vi "Parse VI Documentation String.vi"(5 "LANG ID":string="CＮ", 7 "NOTE-Map":variant, 11 "Documentation":string) -> (0 "Ctrl-Doc Map":variant, 1 "Control Docs":cluster{"filtered array":string[]}[](array[cluster]), 2 "Core Doc":string, 3 "Documentation (Dup)":string, 4 "OUTPUT":string, 6 "INPUT":string)   [LabVIEW 2017, in "csmdoc.lvlib"]
doc: "### Parse VI Documentation String.vi\n\n-- <b>Controls</b> --\n- <b>NOTE-Map</b>:\n- <b>Documentation</b>:\n\n-- <b>Indicators</b> --\n- <b>Ctrl-Doc Map</b>:\n- <b>Control Docs</b>:\n- <b>Core Doc</b>:\n- <b>Documentation (dup)</b>:"
uses:
  csmdoc.lvlib
  _tool/_file/csm-file-support.lvlib
  Communicable State Machine.lvlib
  _Shared/CSM Shared.lvlib
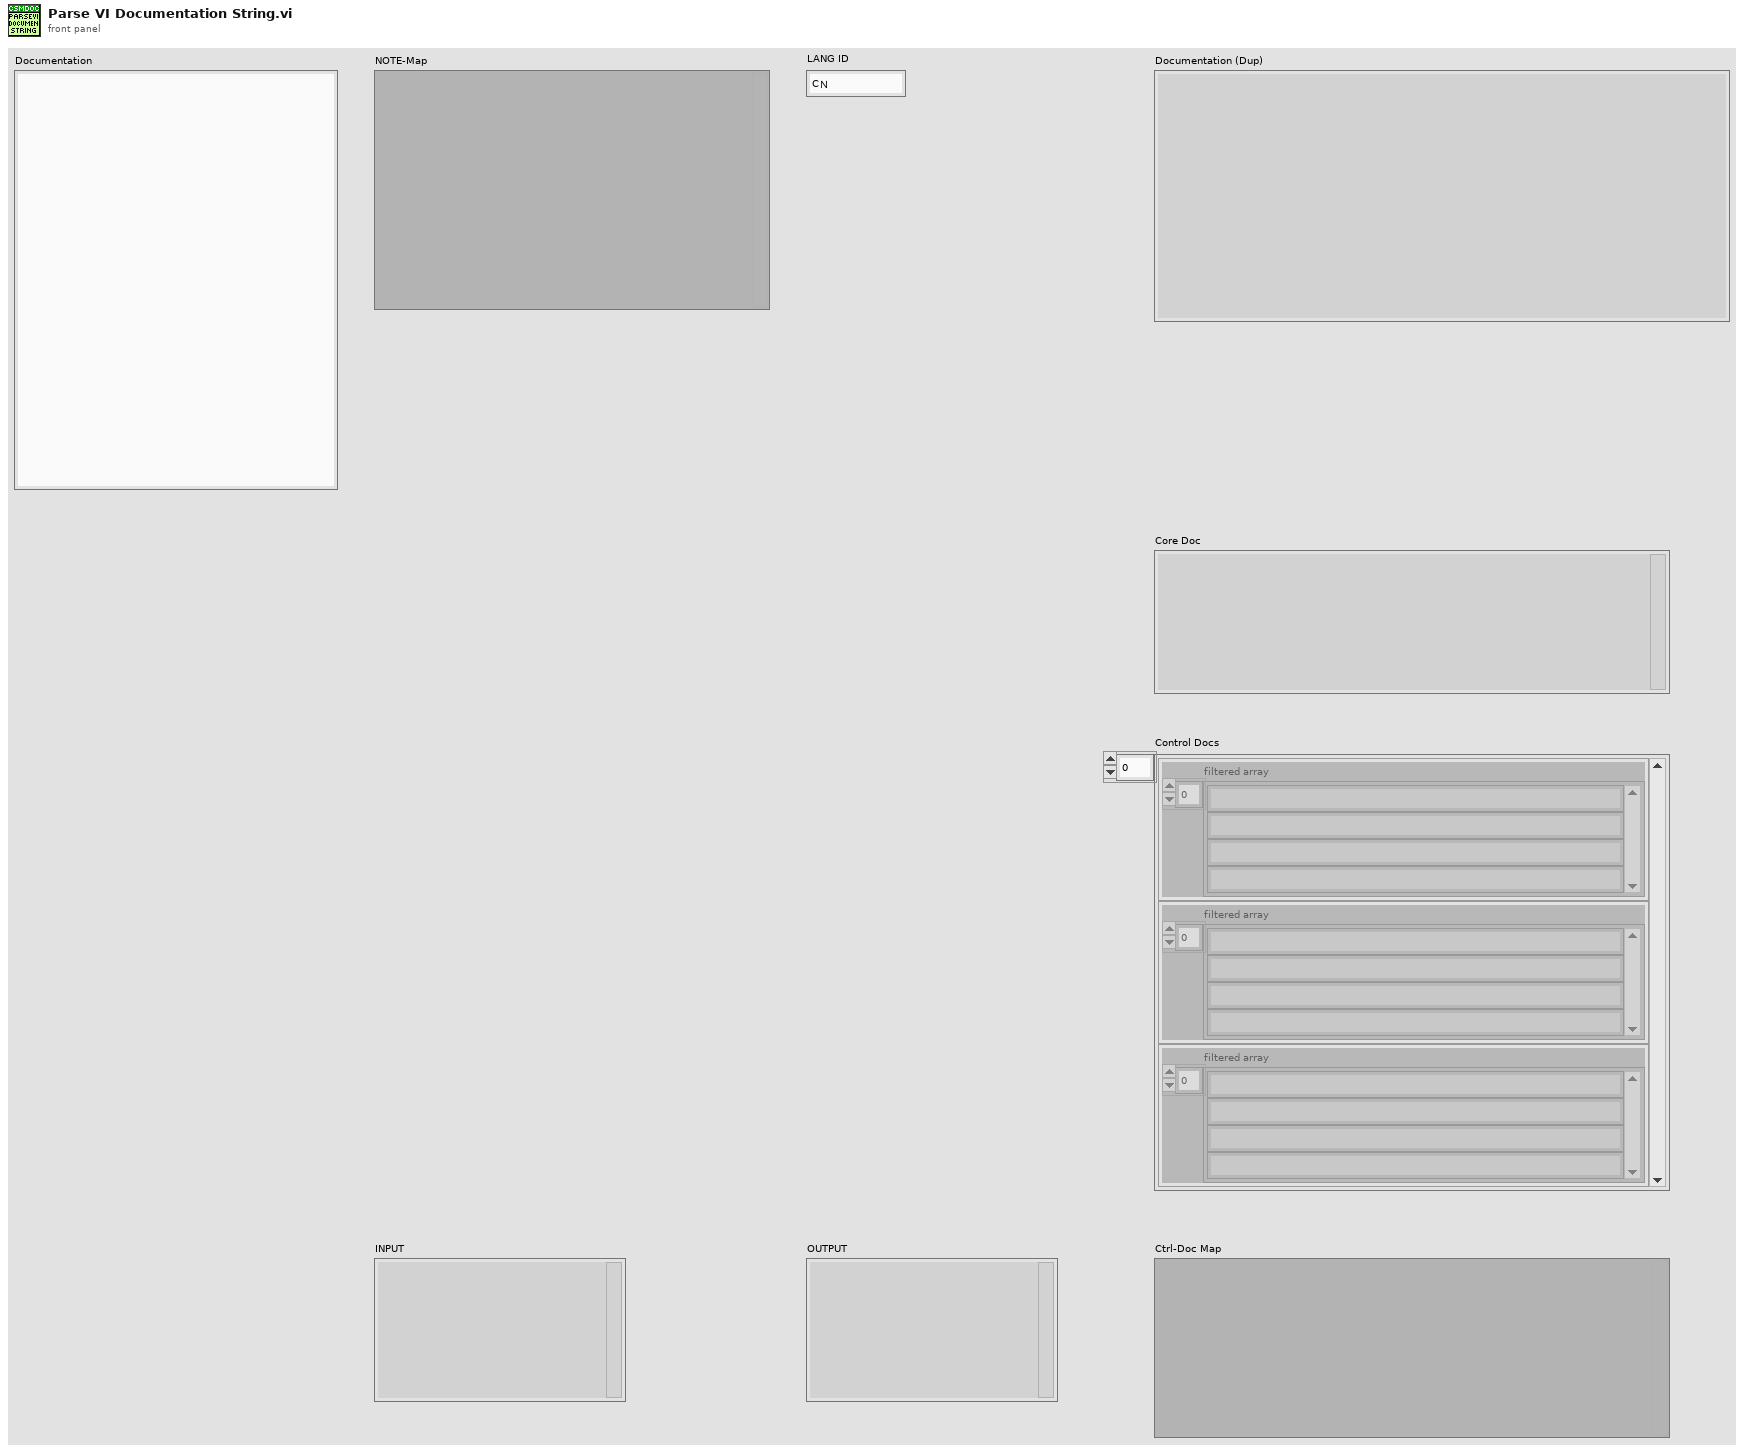
[diagram p1: front panel]
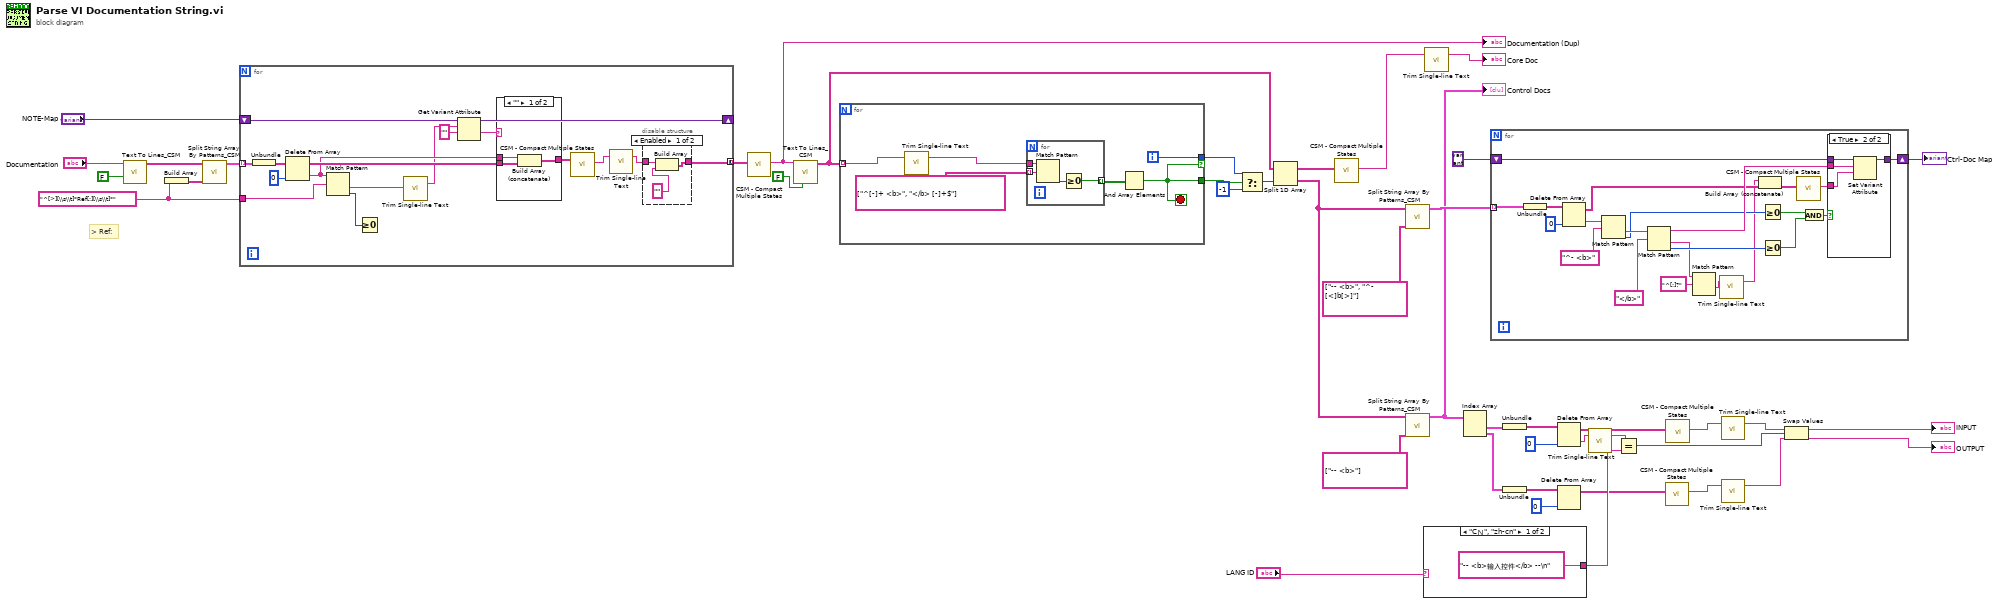
[diagram p0: block diagram]
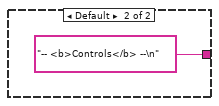
[diagram p2: hidden frame]
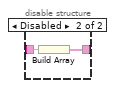
[diagram p4: hidden frame]
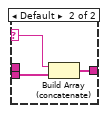
[diagram p5: hidden frame]
diagram:
  w28 = "^[>][\\s\\t]*Ref[:][\\s\\t]*" ("delimited string")
  # "> Ref:"
  n1 = call "Text To Lines_CSM.vi"("Remove Empty Lines? (T)"=FALSE ("Remove Empty Lines?(T)"), "String"="Documentation") -> ("Lines"=w30:string[])  [unwired: 8 in, 1 out]
  n2 = Build Array(w28) -> (w31:string[])
  n3 = call "Split String Array By Patterns_CSM.vi"("Patterns"=w31, "Text Array"=w30) -> ("Array"=w29:cluster{"filtered array":string[]}[])  [unwired: 9 in]
  n4 = for {
    tunnel: w29 -> [w61] mode=indexing
    tunnel: w28 -> [w58]
    shift-right: [w54] -> _
    shift-left: "NOTE-Map" -> [w55]
    tunnel: [w52] -> w26 mode=concatenating
    n5 = Unbundle(w61) -> ("filtered array"=w60:string[])
    n6 = Delete From Array(array=w60, index=0) -> (deleted portion=w53:string, array with subset deleted=w56:string[])  [unwired: 1 in]
    n7 = Match Pattern(string=w53, regular expression=w58) -> (after substring=w57:string, offset past match=w51:i32)  [unwired: 1 in, 2 out]
    n8 = Greater Or Equal To 0?(x=w51) -> ()  [unwired: 1 out]
    n9 = call "Trim Single-line Text.vi"("single-line text"=w57) -> ("trimed text"=w50:string)  [unwired: 2 in]
    n10 = Get Variant Attribute(Variant=w55, name=w50, default value (empty Variant)="" ("delimited string")) -> (duplicate Variant=w54:variant, value=w46:string)  [unwired: 1 in, 2 out]
    n11 = case shown="\"\"" w46 {
      selector: w46 -> [_ w70]
      tunnel: w56 -> [w69 w72]
      tunnel: [w68 w71] -> w48
      tunnel: w53 -> [w67 _]
      frame "" {
        n12 = Build Array (concatenate)(w67, w69) -> (w68:string[])
      }
      frame Default {
        n13 = Build Array (concatenate)(w70, w72) -> (w71:string[])
      }
    }
    n14 = call "CSM - Compact Multiple States.vi"("Multiple States"=w48) -> ("States"=w47:string)  [unwired: 9 in]
    n15 = call "Trim Single-line Text.vi"("single-line text"=w47) -> ("trimed text"=w45:string)  [unwired: 2 in]
    n16 = disable-structure shown="Enabled" {
      disable-tunnel: w45 -> [w64 w66]
      disable-tunnel: [w63 w65] -> w52
      frame Enabled {
        n17 = Build Array(w64, "" ("delimited string")) -> (w63:string[])
      }
      frame Disabled {
        n18 = Build Array(w66) -> (w65:string[])
      }
    }
  }
  n19 = call "CSM - Compact Multiple States.vi"("Multiple States"=w26) -> ("States"=w25:string)  [unwired: 9 in]
  "Documentation (Dup)" <- w25
  n20 = call "Text To Lines_CSM.vi"("Remove Empty Lines? (T)"=FALSE ("Remove Empty Lines?(T)"), "String"=w25) -> ("Lines"=w37:string[])  [unwired: 8 in, 1 out]
  n21 = for {
    tunnel: w37 -> [w78] mode=indexing
    tunnel: [w75] -> w35 if=w73
    tunnel: [w73] -> w34
    i -> [w75]
    stop <- w73 stop-if-true
    n22 = call "Trim Single-line Text.vi"("single-line text"=w78) -> ("trimed text"=w76:string)  [unwired: 2 in]
    n23 = for {
      tunnel: string[] ["^[-]+ <b>", "</b> [-]+$"] ("regular expression") -> [w82] mode=indexing
      tunnel: w76 -> [w81]
      tunnel: [w79] -> w74 mode=indexing
      n24 = Match Pattern(string=w81, regular expression=w82) -> (offset past match=w80:i32)  [unwired: 1 in, 3 out]
      n25 = Greater Or Equal To 0?(x=w80) -> (x >= 0?=w79:bool)
    }
    n26 = And Array Elements(Boolean array=w74) -> (logical AND=w73:bool)
  }
  n27 = Select(t=w35, s=w34, f=-1) -> (s? t:f=w38:i32)
  n28 = Split 1D Array(array=w37, index=w38) -> (first subarray=w43:string[], second subarray=w21:string[])
  n29 = call "CSM - Compact Multiple States.vi"("Multiple States"=w43) -> ("States"=w33:string)  [unwired: 9 in]
  n30 = call "Split String Array By Patterns_CSM.vi"("Patterns"=string[] ["-- <b>", "^- [<]b[>]"] ("patterns"), "Text Array"=w21) -> ("Array"=w40:cluster{"filtered array":string[]}[])  [unwired: 9 in]
  n31 = call "Split String Array By Patterns_CSM.vi"("Patterns"=string[] ["-- <b>"] ("patterns"), "Text Array"=w21) -> ("Array"=w20:cluster{"filtered array":string[]}[])  [unwired: 9 in]
  "Control Docs" <- w20
  n32 = case shown="\"CＮ\", \"zh-cn\"" "LANG ID" {
    tunnel: ["-- <b>输入控件</b> --\n" ("string") "-- <b>Controls</b> --\n" ("string")] -> w13
    frame "CＮ", "zh-cn" {
    }
    frame Default {
    }
  }
  n33 = call "Trim Single-line Text.vi"("single-line text"=w33) -> ("trimed text"=→"Core Doc":string)  [unwired: 2 in]
  n34 = Index Array(array=w20) -> (element #1=w17:cluster{"filtered array":string[]}, element #2=w12:cluster{"filtered array":string[]})  [unwired: 2 in]
  n35 = for {
    tunnel: w40 -> [w106] mode=indexing
    shift-right: [w99] -> w42
    shift-left: variant -> [w100]
    n36 = Unbundle(w106) -> ("filtered array"=w85:string[])
    n37 = Delete From Array(array=w85, index=0) -> (deleted portion=w104:string, array with subset deleted=w92:string[])  [unwired: 1 in]
    n38 = Match Pattern(string=w104, regular expression="^- <b>" ("delimited string")) -> (after substring=w102:string, offset past match=w96:i32)  [unwired: 1 in, 2 out]
    n39 = Match Pattern(string=w102, regular expression="</b>" ("delimited string")) -> (before substring=w98:string, after substring=w89:string, offset past match=w95:i32)  [unwired: 1 in, 1 out]
    n40 = Match Pattern(string=w89, regular expression="^[:]?") -> (after substring=w87:string)  [unwired: 1 in, 3 out]
    n41 = call "Trim Single-line Text.vi"("single-line text"=w87) -> ("trimed text"=w86:string)  [unwired: 2 in]
    n42 = Build Array (concatenate)(w86, w92) -> (w90:string[])
    n43 = Greater Or Equal To 0?(x=w96) -> (x >= 0?=w94:bool)
    n44 = Greater Or Equal To 0?(x=w95) -> (x >= 0?=w93:bool)
    n45 = call "CSM - Compact Multiple States.vi"("Multiple States"=w90) -> ("States"=w91:string)  [unwired: 9 in]
    n46 = And(x=w94, y=w93) -> (x .and. y?=w97:bool)
    n47 = case shown="True" w97 {
      tunnel: w100 -> [w107 w111]
      tunnel: [w107 w110] -> w99
      tunnel: w98 -> [_ w109]
      tunnel: w91 -> [_ w108]
      frame False {
      }
      frame True {
        n48 = Set Variant Attribute(Variant=w111, name=w109, value=w108) -> (Variant out=w110:variant)  [unwired: 1 in, 2 out]
      }
    }
  }
  "Ctrl-Doc Map" <- w42
  n49 = Unbundle(w17) -> ("filtered array"=w19:string[])
  n50 = Unbundle(w12) -> ("filtered array"=w9:string[])
  n51 = Delete From Array(array=w19, index=0) -> (deleted portion=w16:string, array with subset deleted=w11:string[])  [unwired: 1 in]
  n52 = Delete From Array(array=w9, index=0) -> (array with subset deleted=w8:string[])  [unwired: 1 in, 1 out]
  n53 = call "Trim Single-line Text.vi"("single-line text"=w16) -> ("trimed text"=w14:string)  [unwired: 2 in]
  n54 = Equal?(x=w14, y=w13) -> (x = y?=w5:bool)
  n55 = call "CSM - Compact Multiple States.vi"("Multiple States"=w8) -> ("States"=w6:string)  [unwired: 9 in]
  n56 = call "CSM - Compact Multiple States.vi"("Multiple States"=w11) -> ("States"=w7:string)  [unwired: 9 in]
  n57 = call "Trim Single-line Text.vi"("single-line text"=w7) -> ("trimed text"=w2:string)  [unwired: 2 in]
  n58 = call "Trim Single-line Text.vi"("single-line text"=w6) -> ("trimed text"=w1:string)  [unwired: 2 in]
  n59 = Swap Values(12:w2, 13:w5, 14:w1) -> (1:→"INPUT":string, 3:→"OUTPUT":string)
